vi "Pulse Attribute, Find Stimulus Polarity.vi"(8 "error in":errorcluster, 9 "amp min":dbl=-2.3038735826160917 format="%.4f", 10 "amp max":dbl=2.633932511936763 format="%.4f", 11 "waveform":waveform(dbl)={"t0"=timestamp(3473168073.631 s since 1904-01-01), "dt"=1e-08, "Y"=[], "attributes"=variant("Average Size"=variant(dbl 15.0), "NSamp"=variant(dbl 400000.0), "Resistance (ohms)"=variant(dbl 500.0), "Samp Freq (MHz)"=variant(dbl 100.0), "dt (us)"=variant(dbl 0.01))}) -> (0 "error out":errorcluster, 1 "Recvy Amp":dbl=nan format="%.4f", 2 "Stim Amp":dbl=nan format="%.4f", 3 "waveform out":waveform(dbl)={"t0"=timestamp(-9593225999.921999 s since 1904-01-01), "dt"=nan, "Y"=[]})   [LabVIEW 2010]
doc: "This function calculates the Stimulus Trigger (s) and Recovery Trigger (s) instants; and adjusts the polarity of the Stimulus Amplitude and Recovery Amplitude for a bipolar pulse waveform. The trigger results are stored as Waveform attributes in double precision floating point format.\n\nThe Stimulus Trigger is the First Transition Occurrence Instant. The Recovery Trigger is the Third Transition Occurrence Instant. (IEEE Standard 181-2003, Standard on Transitions, Pulses, and Related Waveforms)\n\nThe trigger point levels are consistent with the pulse duration triggers. Pulse duration is measured between the points on the pulse equal to one-third of the pulse amplitude. (EN 45502-2-1:2003 Active Implant Medical Devices - Part 2-1, Measurement of implantable pulse generator and lead characteristics)\n\nIf \"error in\" is TRUE, or a trigger can't be calculated, the result is set to NaN."
uses:
  <vilib>/measure/mamon.llb/Trigger Detection for 1 Channel.vi
  <vilib>/measure/NI_MAPro.lvlib
panel:
  in  "hysteresis":dbl format="%.3f"
  out "Recvy Trigger (s)":dbl=nan format="%.3p"
  out "Stim Trigger (s)":dbl=nan format="%.3p"
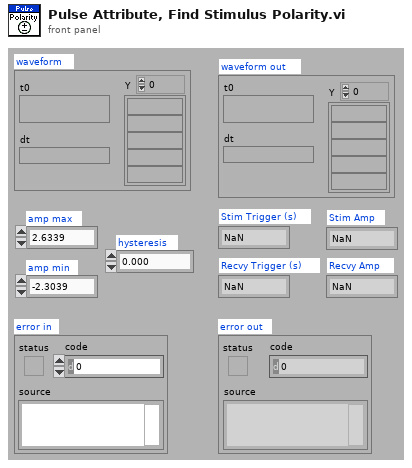
[diagram p1: front panel]
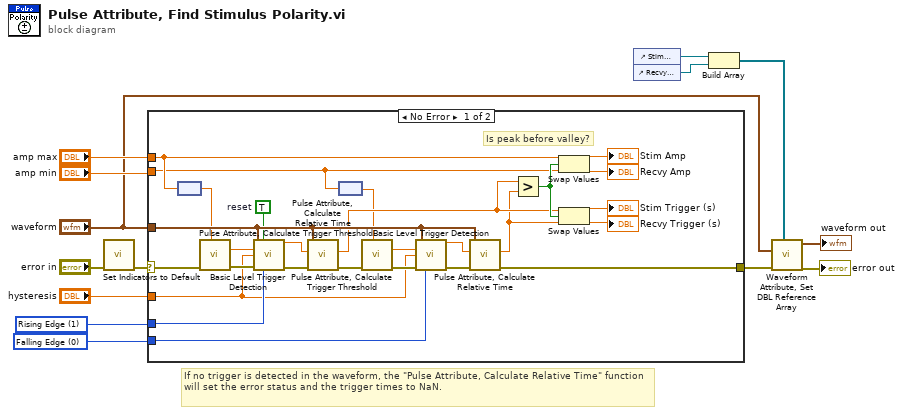
[diagram p0: block diagram]
diagram:
  w4 = u16 0 items=["Falling Edge", "Rising Edge"] ("trigger slope")
  w5 = u16 1 items=["Falling Edge", "Rising Edge"] ("trigger slope")
  # "If no trigger is detected in the waveform, the \"Pulse Attribute, Calculate Relative Time\" function will set the error status and the trigger times to NaN."
  n1 = call "Set Indicators to Default.vi"("error in"="error in") -> ("error out"=w1:errorcluster)  [unwired: 6 in]
  n2 = case shown="No Error" w1 {
    selector: w1 -> [w38 w42]
    tunnel: "amp max" -> [w17 _]
    tunnel: "waveform" -> [w28 _]
    tunnel: [w33 w42] -> w10
    tunnel: "amp min" -> [w15 _]
    tunnel: w5 -> [w41 _]
    tunnel: w4 -> [w40 _]
    tunnel: "hysteresis" -> [w24 _]
    frame No Error {
      w19 = TRUE  # reset
      # "Is peak before valley?"
      n3 = node(w17) -> (w18:dbl[unit])
      n4 = call "Pulse Attribute, Calculate Trigger Threshold.vi"("pulse amp"=w18, "error in"=w38) -> ("error out"=w39:errorcluster, "trigger level (V)"=w37:dbl)  [unwired: 5 in]
      n5 = call-poly <vilib>:"Basic Level Trigger Detection.vi"("signal in"=w28, "reset"=w19, "level"=w37, "hysteresis"=w24, "error in (no error)"=w39, "trigger slope"=w41) -> ("trigger location"=w30:dbl, "error out"=w32:errorcluster)  [unwired: 7 in, 1 out]
      n6 = call "Pulse Attribute, Calculate Relative Time.vi"("error in"=w32, "index"=w30, "waveform"=w28) -> ("error out"=w31:errorcluster, "relative time (s)"=w27:dbl)  [unwired: 4 in, 1 out]
      n7 = node(w15) -> (w16:dbl[unit])
      n8 = call "Pulse Attribute, Calculate Trigger Threshold.vi"("pulse amp"=w16, "error in"=w31) -> ("error out"=w35:errorcluster, "trigger level (V)"=w36:dbl)  [unwired: 5 in]
      n9 = call-poly <vilib>:"Basic Level Trigger Detection.vi"("signal in"=w28, "level"=w36, "hysteresis"=w24, "error in (no error)"=w35, "trigger slope"=w40) -> ("trigger location"=w26:dbl, "error out"=w29:errorcluster)  [unwired: 8 in, 1 out]
      n10 = call "Pulse Attribute, Calculate Relative Time.vi"("error in"=w29, "index"=w26, "waveform"=w28) -> ("error out"=w33:errorcluster, "relative time (s)"=w25:dbl)  [unwired: 4 in, 1 out]
      n11 = Greater?(x=w27, y=w25) -> (0:w34:bool)
      n12 = Swap Values(12:w17, 13:w34, 14:w15) -> (1:→"Stim Amp":dbl, 3:→"Recvy Amp":dbl)
      n13 = Swap Values(12:w27, 13:w34, 14:w25) -> (1:→"Stim Trigger (s)":dbl, 3:→"Recvy Trigger (s)":dbl)
    }
    frame Error {
    }
  }
  n14 = control-ref of="Stim Trigger (s)"() -> (w7:refnum<vi>)
  n15 = control-ref of="Recvy Trigger (s)"() -> (w6:refnum<vi>)
  n16 = Build Array(w7, w6) -> (w8:refnum<vi>[])
  n17 = call "Waveform Attribute, Set DBL Reference Array.vi"("Refnum Array"=w8, "error in"=w10, "waveform"="waveform") -> ("error out"=→"error out":errorcluster, "waveform out"=→"waveform out":waveform(dbl))  [unwired: 5 in]
